vi "GetImpairReports.vi"(8 "error in (no error)":errorcluster, 11 "C37BehaviourPlugin in":refnum<class "C37BehaviourPlugin.lvclass">) -> (0 "error out":errorcluster, 3 "C37BehaviourPlugin out":refnum<class "C37BehaviourPlugin.lvclass">)   [LabVIEW 2014, in "PmuImpairPlugins.lvlib" / "C37BehaviourPlugin.lvclass"]
uses:
  C37BehaviourPlugin.lvclass
  PmuImpairPluginBase_class/PmuImpairPluginBase.lvclass/PmuImpairPluginBase.ctl
  EventPlugins/EventPluginBaseClass/TypeDefs/clEvtReport.ctl
  PmuImpairPluginBase_class/Accessors/Read clEvtConfig.vi
  PmuImpairPluginBase_class/Accessors/Read BusNumber.vi
  PmuImpairPluginBase_class/Accessors/Read dblImpairParams.vi
  PmuImpairPluginBase_class/Accessors/Read clImpairConfig.vi
  EventPlugins/EventPluginBaseClass/EventPluginBaseClass.lvclass
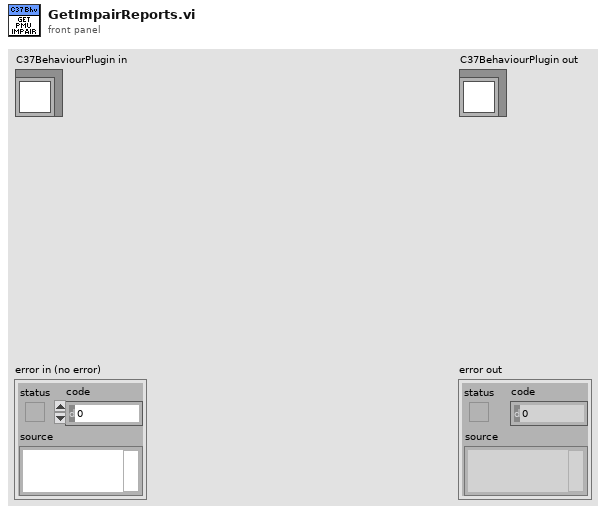
[diagram p1: front panel]
types:
  T1 = typedef "EventPlugins.lvlib/EventPluginBaseClass.lvclass/clEvtReport.ctl" = cluster{"Timestamp":dbl, "Synx":cdb[], "Freq":dbl, "ROCOF":dbl, "ID":i16}
  T2 = typedef "PmuImpairPlugins.lvlib/PmuImpairPluginBase.lvclass/clImpairConfig.ctl" = cluster{"FilterType":string, "bPosSeq":bool}
  T3 = typedef "EventPlugins.lvlib/EventPluginBaseClass.lvclass/clEvtConfig.ctl" = cluster{"T0(UTC)":dbl, "F0":dbl, "Fs":i32, "FSamp":u32, "bPosSeq":bool}
  T4 = typedef "EventPlugins.lvlib/EventPluginBaseClass.lvclass/clEvtReportArray.ctl" = T1[]
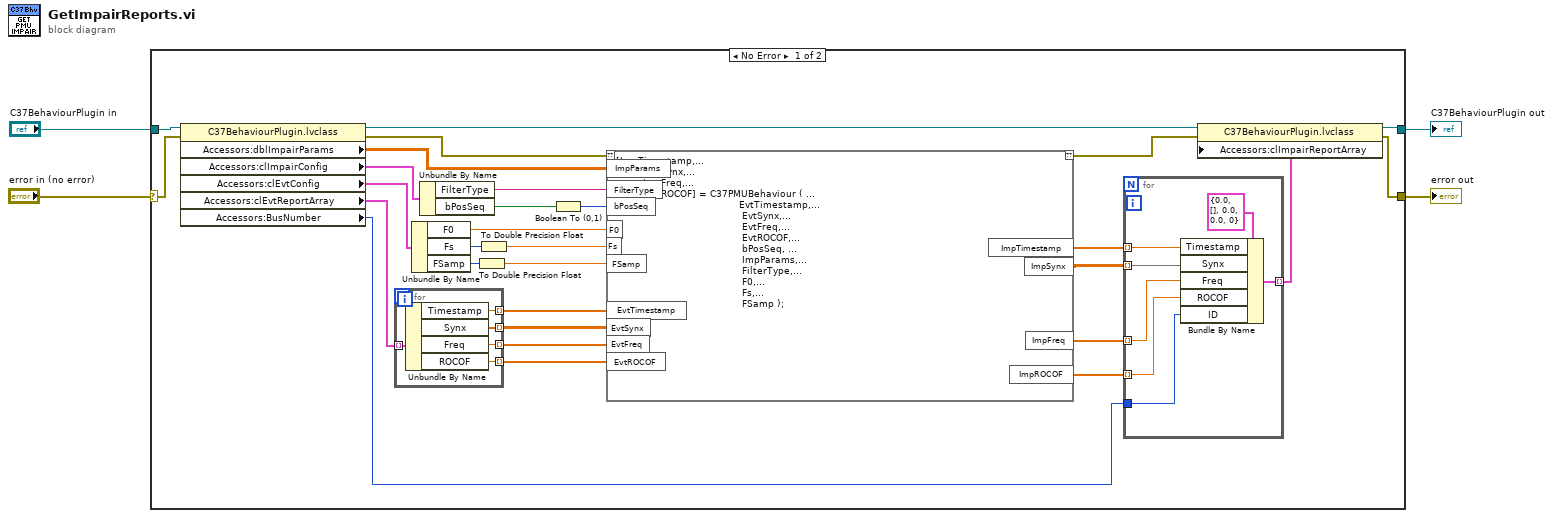
[diagram p0: block diagram]
diagram:
  n1 = case shown="No Error" "error in (no error)" {
    selector: "error in (no error)" -> [w33 w47]
    tunnel: [w12 w47] -> w3
    tunnel: [w13 w46] -> w1
    tunnel: "C37BehaviourPlugin in" -> [w17 w46]
    frame No Error {
      n2 = property class="C37BehaviourPlugin.lvclass"(reference=w17, error in=w33) -> (reference out=w14:refnum<class "C37BehaviourPlugin.lvclass">, error out=w32:errorcluster, "Accessors:dblImpairParams"=w6:dbl[][], "Accessors:clImpairConfig"=w10:T2, "Accessors:clEvtConfig"=w9:T3, "Accessors:clEvtReportArray"=w8:T4, "Accessors:BusNumber"=w7:u8)
      n3 = for {
        tunnel: w8 -> [w45] mode=indexing
        tunnel: [w44] -> w27 mode=indexing
        tunnel: [w43] -> w26 mode=indexing
        tunnel: [w42] -> w25 mode=indexing
        tunnel: [w41] -> w18 mode=indexing
        n4 = Unbundle By Name(w45) -> ("Timestamp"=w41:dbl, "Synx"=w44:cdb[], "Freq"=w43:dbl, "ROCOF"=w42:dbl)
      }
      n5 = Unbundle By Name(w9) -> ("F0"=w30:dbl, "Fs"=w29:i32, "FSamp"=w28:u32)
      n6 = Unbundle By Name(w10) -> ("FilterType"=w31:string, "bPosSeq"=w11:bool)
      n7 = To Double Precision Float(number=w28) -> (double precision float=w23:dbl)
      n8 = To Double Precision Float(number=w29) -> (double precision float=w24:dbl)
      n9 = Boolean To (0,1)(Boolean=w11) -> (0, 1=w5:i16)
      n10 = script code="[ImpTimestamp,...\n         ImpSynx,...\n         ImpFreq,...\n         ImpROCOF] = C37PMUBehaviour ( ...\n                                         EvtTimestamp,...\n                                          EvtSynx,...\n                                          EvtFreq,...\n                                          EvtROCOF,...\n                                          bPosSeq, ...\n                                          ImpParams,...\n                                          FilterType,...\n                                          F0,...\n                                          Fs,...\n                                          FSamp );"("??"=w32, "ImpParams"=w6, "FilterType"=w31, "bPosSeq"=w5, "F0"=w30, "Fs"=w24, "FSamp"=w23, "EvtTimestamp"=w18, "EvtSynx"=w27, "EvtFreq"=w26, "EvtROCOF"=w25) -> ("??"=w16:errorcluster, "ImpTimestamp"=w22:dbl[], "ImpSynx"=w21:cdb[][], "ImpFreq"=w20:dbl[], "ImpROCOF"=w19:dbl[])
      n11 = for {
        tunnel: w22 -> [w39] mode=indexing
        tunnel: w21 -> [w38] mode=indexing
        tunnel: w20 -> [w36] mode=indexing
        tunnel: w19 -> [w35] mode=indexing
        tunnel: [w37] -> w15 mode=indexing
        tunnel: w7 -> [w34]
        n12 = Bundle By Name(cluster=T1 {"Timestamp"=0.0, "Synx"=[], "Freq"=0.0, "ROCOF"=0.0, "ID"=0} ("clEvtReport"), "Timestamp"=w39, "Synx"=w38, "Freq"=w36, "ROCOF"=w35, "ID"=w34) -> (w37:T1)
      }
      n13 = property class="C37BehaviourPlugin.lvclass"(reference=w14, error in=w16, "Accessors:clImpairReportArray"=w15) -> (reference out=w13:refnum<class "C37BehaviourPlugin.lvclass">, error out=w12:errorcluster)
    }
    frame Error {
    }
  }
  "error out" <- w3
  "C37BehaviourPlugin out" <- w1
